vi "WriteAll.vi"(6 "myBool":bool, 8 "error in (no error)":errorcluster, 9 "someNumber":dbl, 10 "anotherNumber":dbl, 11 "Class4 in":refnum<class "Class4.lvclass">) -> (0 "error out":errorcluster, 3 "Class4 out":refnum<class "Class4.lvclass">)   [LabVIEW 2020, in "Class4.lvclass"]
doc: "GCraftsman JSON Object Serialization Toolkit\nwww.GCraftsman.com\nCopyright (c) 2017, GCraftsman"
uses:
  Class4.lvclass
  Class4.lvclass/Class4.ctl
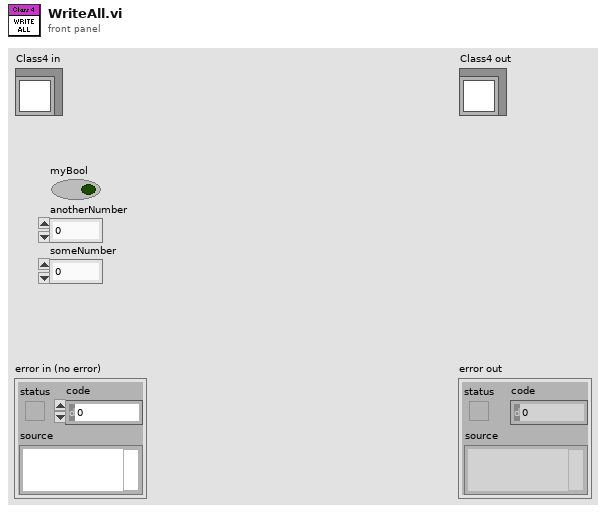
[diagram p1: front panel]
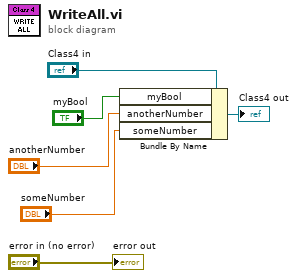
[diagram p0: block diagram]
diagram:
  n1 = Bundle By Name(cluster="Class4 in", "myBool"="myBool", "anotherNumber"="anotherNumber", "someNumber"="someNumber") -> (→"Class4 out":refnum<class "Class4.lvclass">)
  "error out" <- "error in (no error)"
